vi "Window-Enter funct trig width.vi"(8 "error in (no error)":errorcluster) -> (0 "error out":errorcluster)   [LabVIEW 2013]
doc: "Use this template to create a dialog box with event handling."
uses:
  <vilib>/Utility/miscctls.llb/LVPointTypeDef.ctl
  ROI Entry screen/Globals/gl_ROI Entry UI globals.vi
  Global Variables/General Globals.vi
  Global Variables/FPGAstatus_Reference.vi
panel:
  in  "Pulse Width":dbl=0.1 min=0.01 max=0.01 step=0.1 format="%#.2f ms"
  in  "OK":bool
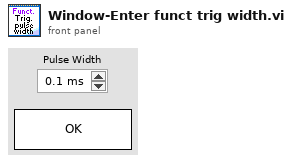
[diagram p1: front panel]
types:
  T1 = typedef "LVPointTypeDef.ctl" = cluster{"Horizontal":i16, "Vertical":i16}
  T2 = typedef "ROI entry screen ctrl refs cluster.ctl" = cluster{"Done button":refnum<vi>, "Imaging button":refnum<vi>, "Acquisition button":refnum<vi>, "POI dwell time (us)":refnum<vi>, "Scan dwell time per pixel (us)":refnum<vi>, "# of planes":refnum<vi>, "Zoom":refnum<vi>, "Equal size":refnum<vi>, "Channel":refnum<vi>, "Image Display":refnum<vi>, "Z-Plane Selector":refnum<vi>, "Number of lines left":refnum<vi>, "Z-stack folder path":refnum<vi>, "POI Density":refnum<vi>, "Arb Plane Entry":refnum<vi>, "Whole plane":refnum<vi>, "Clear Last":refnum<vi>, "Clear All":refnum<vi>, "Trial Length (sec)":refnum<vi>, "Palette Type":refnum<vi>, "Intensity slider":refnum<vi>, "# POI":refnum<vi>, "Max Z Proj":refnum<vi>, "Zplane ind":refnum<vi>, "Wavelength (nm)":refnum<vi>, "Number of Trials":refnum<vi>, "Funct stim.trig.enable":refnum<vi>, "Funct stim.trig.delay (s)":refnum<vi>, "Line Mode":refnum<vi>, "Step size (µm)":refnum<vi>, "ROI move mode":refnum<vi>, "Cool-down time (s)":refnum<vi>, "Enable cool-down time":refnum<vi>, "Motor Z ind. (um)":refnum<vi>, "AOL Z ind. (um)":refnum<vi>}
  T3 = typedef "FPGA Ref.ctl" = refnum<k20>
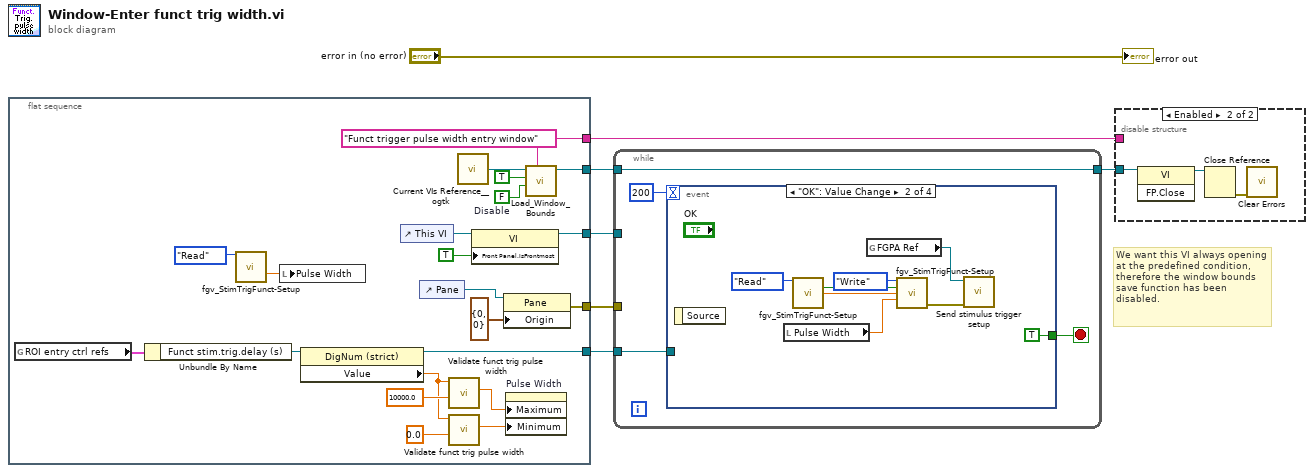
[diagram p0: block diagram]
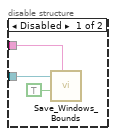
[diagram p2: hidden frame]
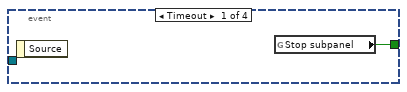
[diagram p3: hidden frame]
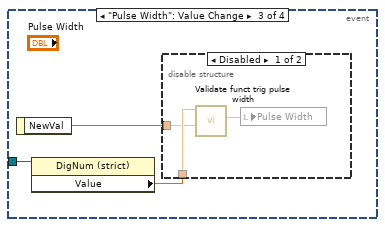
[diagram p4: hidden frame]
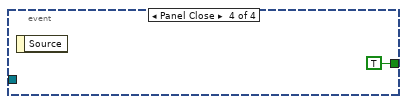
[diagram p6: hidden frame]
diagram:
  # "We want this VI always opening at the predefined condition, therefore the window bounds save function has been disabled."
  n1 = flat-sequence {
    tunnel: [w26] -> w7
    tunnel: [w24] -> w6
    tunnel: [w20] -> w5
    tunnel: [w19] -> w4
    tunnel: [w13] -> w1
    frame #0 {
      w21 = FALSE  # Disable
      w20 = "Funct trigger pulse width entry window" ("Window Name (i.e. Key)")
      n2 = global read "gl_ROI Entry UI globals.vi" "ROI entry ctrl refs"() -> (w15:T2)
      n3 = Unbundle By Name(w15) -> ("Funct stim.trig.delay (s)"=w14:refnum<vi>)
      n4 = call "fgv_StimTrigFunct-Setup.vi"("Function"=enum16{"Intialize", "Write", "Read", "Clear"}."Read") -> ("Funct stim.trig.width (ms)"=w17:dbl)  [unwired: 11 in, 3 out]
      n5 = local write "Pulse Width"(w17) -> ()
      n6 = property class="DigNum (strict)"(reference=w14) -> (reference out=w13:refnum<vi>, "Value"=w8:dbl)  [unwired: 1 in, 1 out]
      n7 = control-ref of="This VI"() -> (w27:refnum<vi>)
      n8 = control-ref of="Pane"() -> (w23:refnum<vi>)
      n9 = call "Validate funct trig pulse width.vi"("Requested trigger pulse width (ms)"=10000.0, "Trigger delay (sec)"=w8) -> ("functional acq. stimulus trigger pulse width (ms)"=w10:dbl)  [unwired: 9 in]
      n10 = call "Validate funct trig pulse width.vi"("Requested trigger pulse width (ms)"=0.0, "Trigger delay (sec)"=w8) -> ("functional acq. stimulus trigger pulse width (ms)"=w9:dbl)  [unwired: 9 in]
      n11 = call "Current VIs Reference__ogtk.vi"() -> ("Current VI's reference"=w22:refnum<vi>)  [unwired: 5 in]
      n12 = property on="Property Node" class="VI"(reference=w27, "Front Panel.IsFrontmost"=TRUE ("Front Panel Window:Is Frontmost")) -> (reference out=w26:refnum<vi>)  [unwired: 1 in, 1 out]
      n13 = property class="Pane"(reference=w23, "Origin"=T1 {"Horizontal"=0, "Vertical"=0}) -> (error out=w24:errorcluster)  [unwired: 1 in, 1 out]
      n14 = property on="Pulse Width" class="DigNum (strict)"("Maximum"=w10, "Minimum"=w9) -> ()  [unwired: 2 in, 2 out]
      n15 = call "Load_Window_Bounds.vi"("Window Name (i.e. Key)"=w20, "Disable"=w21, "First Call"=TRUE, "Window VI's Ref"=w22) -> ("reference out"=w19:refnum<vi>)  [unwired: 4 in, 3 out]
    }
  }
  n16 = while {
    tunnel: w6 -> [_]
    tunnel: w7 -> [_]
    tunnel: w4 -> [w30]
    tunnel: [w30] -> w3
    tunnel: w1 -> [w29]
    stop <- w32 stop-if-true
    n17 = event shown="[1] \"OK\": Value Change" {
      selector: _ -> [_ _ _ _]
      dyn-events: _ -> [_ _ _ _]
      timeout: 200 -> [_ _ _ _]
      tunnel: [w33 TRUE ("Stop?") _ TRUE ("Stop?")] -> w32
      tunnel: w29 -> [_ _ w44 _]
      event Timeout {
        n18 = event-data() -> ()  [unwired: 1 in, 1 out]
        n19 = global read "General Globals.vi" "Stop subpanel"() -> (w33:bool)
      }
      event "OK": Value Change {
        n20 = event-data() -> ()  [unwired: 1 in, 1 out]
        n21 = local read "Pulse Width"() -> (w34:dbl)
        n22 = call "fgv_StimTrigFunct-Setup.vi"("Function"=enum16{"Intialize", "Write", "Read", "Clear"}."Read") -> ("Live stim.trig.enable"=w38:bool, "Funct stim.trig.delay (sec)"=w37:dbl)  [unwired: 11 in, 2 out]
        n23 = global read "FPGAstatus_Reference.vi" "FGPA Ref"() -> (w36:T3)
        n24 = call "fgv_StimTrigFunct-Setup.vi"("Function"=enum16{"Intialize", "Write", "Read", "Clear"}."Write", "Live stim.trig.enable"=w38, "Funct stim.trig.delay (sec)"=w37, "Funct stim.trig.width (ms)"=w34) -> ("error out"=w35:errorcluster)  [unwired: 8 in, 3 out]
        n25 = call "Send stimulus trigger setup.vi"("error in (no error)"=w35, "FPGA ref in"=w36) -> ()  [unwired: 8 in, 2 out]
      }
      event "Pulse Width": Value Change {
        n26 = event-data() -> ("NewVal"=w42:dbl)  [unwired: 1 in]
        n27 = property class="DigNum (strict)"(reference=w44) -> ("Value"=w43:dbl)  [unwired: 1 in, 2 out]
        n28 = disable-structure shown="Disabled" {
          disable-tunnel: w43 -> [w47 _]
          disable-tunnel: w42 -> [w46 _]
          frame Disabled {
            n29 = call "Validate funct trig pulse width.vi"("Requested trigger pulse width (ms)"=w46, "Trigger delay (sec)"=w47) -> ("functional acq. stimulus trigger pulse width (ms)"=w45:dbl)  [unwired: 9 in]
            n30 = local write "Pulse Width"(w45) -> ()
          }
          frame Enabled {
          }
        }
      }
      event Panel Close {
        n31 = event-data() -> ()  [unwired: 1 in, 1 out]
      }
    }
  }
  n32 = disable-structure shown="Enabled" {
    disable-tunnel: w5 -> [w51 _]
    disable-tunnel: w3 -> [w49 w52]
    frame Disabled {
      n33 = call "Save_Windows_Bounds.vi"("Window Name (i.e. Key)"=w51, "Front Panel Window:Open"=TRUE, "Window VI's Ref"=w49) -> ()  [unwired: 8 in, 1 out]
    }
    frame Enabled {
      n34 = invoke class="VI" method="FP.Close"(reference=w52) -> (reference out=w54:refnum<vi>)  [unwired: 2 in, 2 out]
      n35 = Close Reference(reference=w54) -> (error out=w53:errorcluster)  [unwired: 1 in]
      n36 = call <vilib>:"Clear Errors.vi"("error in (no error)"=w53) -> ()  [unwired: 6 in, 1 out]
    }
  }
  "error out" <- "error in (no error)"
